vi "setFormat.vi"(8 "error in (no error)":errorcluster, 10 "format":T1, 11 "Instrument.VSource in":refnum<class "Instrument.VNA.lvclass">) -> (0 "error out":errorcluster, 3 "Instrument.VSource out":refnum<class "Instrument.VNA.lvclass">)   [LabVIEW 2019, in "Instrument.VNA.lvclass"]
uses:
  Instrument.VNA.lvclass
  Typedefs/VNA.Commands--Enum.ctl
  Typedefs/Format--enum.ctl
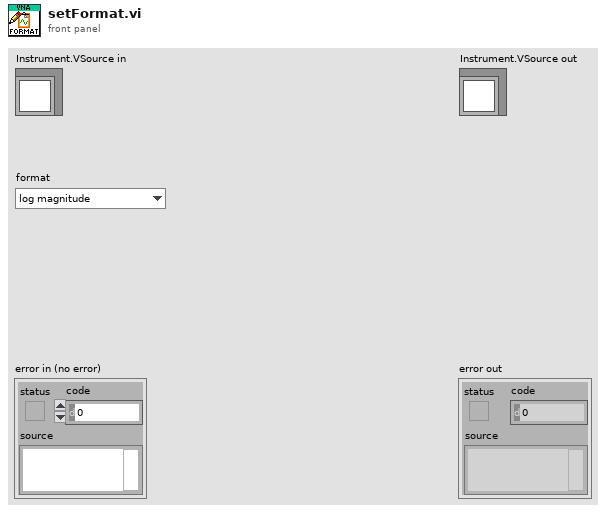
[diagram p1: front panel]
types:
  T1 = typedef "Instrument.VNA.lvclass/Format--enum.ctl" = enum16{"log magnitude", "phase", "delay", "Smith chart", "polar", "linear magnitude", "standing wave ratio", "real", "imaginary"}
  T2 = typedef "Instrument.VNA.lvclass/VNA.Commands--Enum.ctl" = enum16{"getData", "setAverage", "setFormat", "setMeasurement", "setPower", "setSweep"}
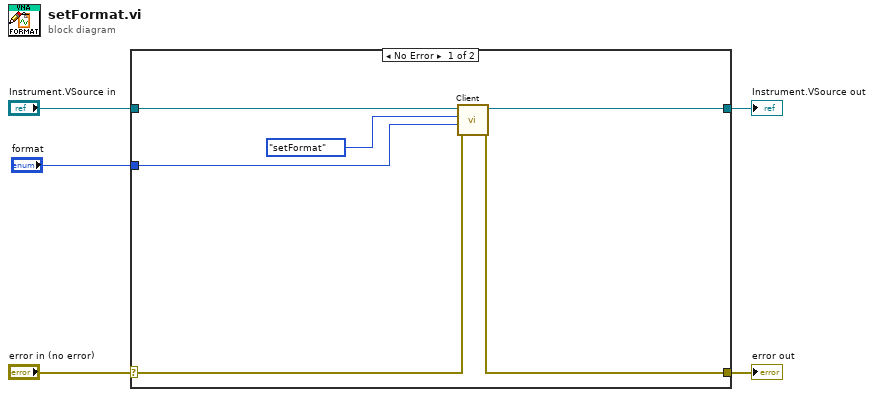
[diagram p0: block diagram]
diagram:
  n1 = case shown="No Error" "error in (no error)" {
    selector: "error in (no error)" -> [w8 w13]
    tunnel: [w10 w13] -> w4
    tunnel: [w11 w12] -> w2
    tunnel: "Instrument.VSource in" -> [w9 w12]
    tunnel: "format" -> [w6 _]
    frame No Error {
      n2 = call-dynamic "Client.vi"("error in (no error)"=w8, "Data in"=w6, "Command in"=VNA.Commands--Enum."setFormat" ("Commands"), "Instrument in"=w9) -> ("error out"=w10:errorcluster, "Instrument out"=w11:refnum<class "Instrument.VNA.lvclass">)  [unwired: 4 in, 2 out]
    }
    frame Error {
    }
  }
  "error out" <- w4
  "Instrument.VSource out" <- w2
